vi "FGV Error Manager.vi"(1 "error_manager in":refnum<class "LogRotate.lvclass">) -> (0 "error_manager out":refnum<class "LogRotate.lvclass">)   [LabVIEW 2019, in "Error_Manager.lvlib" / "LogRotate.lvclass"]
doc: "This method stores error manager object to be able to use it around application"
uses:
  LogRotate.lvclass
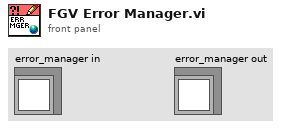
[diagram p1: front panel]
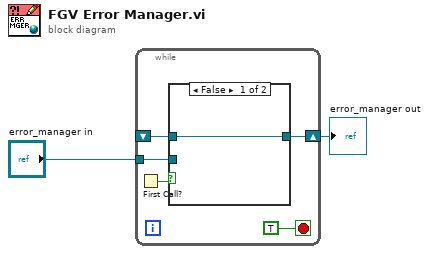
[diagram p0: block diagram]
diagram:
  n1 = while {
    shift-right: [w4] -> w1
    shift-left: _ -> [w5]
    tunnel: "error_manager in" -> [w3]
    stop <- TRUE stop-if-true
    n2 = First Call?() -> (First Call?: T/F=w6:bool)
    n3 = case shown="False" w6 {
      tunnel: w5 -> [w8 _]
      tunnel: [w8 w9] -> w4
      tunnel: w3 -> [_ w9]
      frame False {
      }
      frame True {
      }
    }
  }
  "error_manager out" <- w1
